vi "Get Initial Guess.vi"(6 "State":dbl[][](array[numeric]), 9 "Control":dbl[][](array[numeric]), 10 "Time":dbl[](array[numeric]), 11 "nGrid":dbl) -> (3 "Array":dbl[](array[numeric]))   [LabVIEW 2020]
uses:
  <vilib>/Analysis/1siggen.llb/Ramp Pattern by Samples.vi
  <vilib>/Analysis/NI_AALBase.lvlib
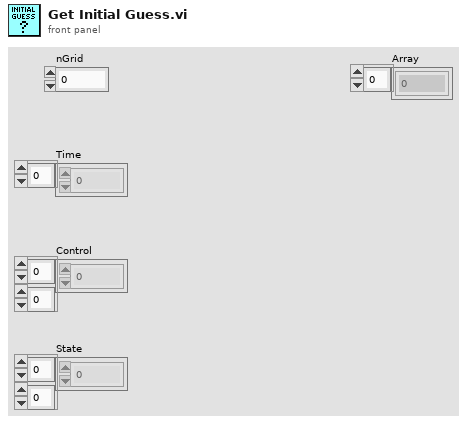
[diagram p1: front panel]
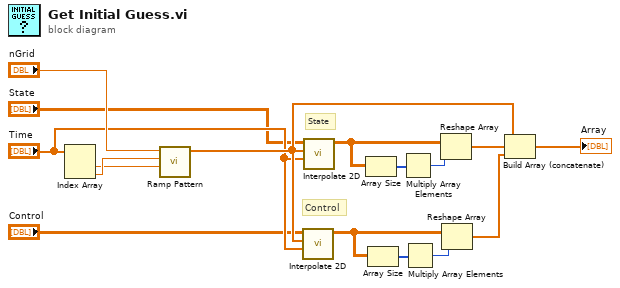
[diagram p0: block diagram]
diagram:
  # "Control"
  # "State"
  n1 = Index Array(array="Time") -> (element #1=w1:dbl, element #2=w2:dbl)  [unwired: 2 in]
  n2 = call-poly <vilib>:"Ramp Pattern.vi"("start"=w1, "end"=w2, "samples"="nGrid") -> ("Ramp Pattern"=w8:dbl[])  [unwired: 7 in, 1 out]
  n3 = call "Interpolate 2D.vi"("X"="Time", "xi"=w8, "2D Array"="Control") -> ("yi"=w13:dbl[][])  [unwired: 8 in]
  n4 = call "Interpolate 2D.vi"("X"="Time", "xi"=w8, "2D Array"="State") -> ("yi"=w9:dbl[][])  [unwired: 8 in]
  n5 = Array Size(array=w9) -> (size(s)=w11:i32[])
  n6 = Array Size(array=w13) -> (size(s)=w12:i32[])
  n7 = Multiply Array Elements(1:w11) -> (0:w10:i32)
  n8 = Multiply Array Elements(1:w12) -> (0:w14:i32)
  n9 = Reshape Array(w9, w10) -> (w7:dbl[])
  n10 = Reshape Array(w13, w14) -> (w6:dbl[])
  n11 = Build Array (concatenate)(w8, w7, w6) -> (→"Array":dbl[])
